vi "compileScript.vi"(8 "error in (no error)":errorcluster, 10 "Path":path, 11 "Compiler in":refnum<class "Compiler.lvclass">) -> (0 "error out":errorcluster, 2 "CompiledList":refnum<class "CompiledList.lvclass">, 3 "Compiler out":refnum<class "Compiler.lvclass">)   [LabVIEW 2011, in "Compiler.lvlib" / "Compiler.lvclass"]
uses:
  Compiler.lvclass
  CompiledList/CompiledList.lvclass
  Compiler.lvclass/Compiler.ctl
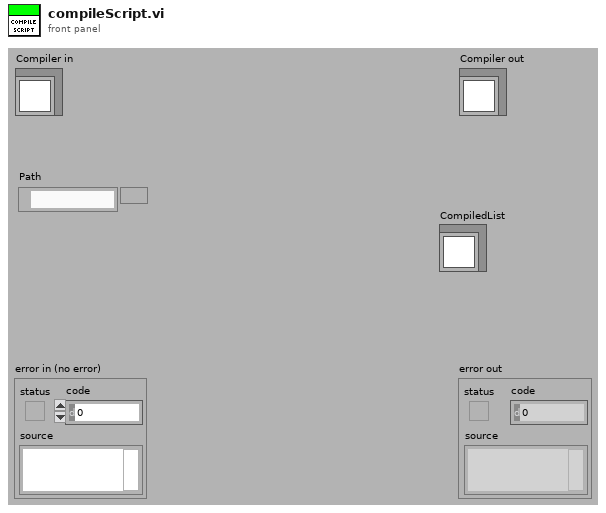
[diagram p1: front panel]
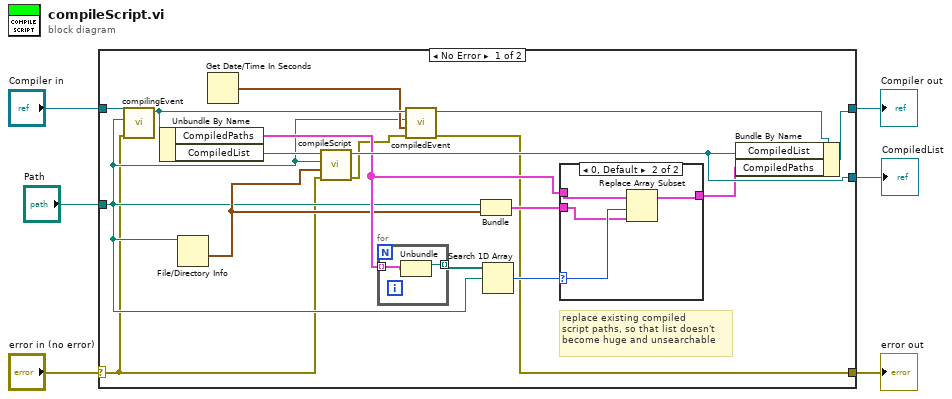
[diagram p0: block diagram]
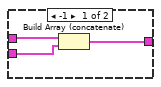
[diagram p2: hidden frame]
diagram:
  n1 = case shown="No Error" "error in (no error)" {
    selector: "error in (no error)" -> [w10 w34]
    tunnel: [w9 w34] -> w5
    tunnel: [w7 w33] -> w3
    tunnel: "Compiler in" -> [w16 w33]
    tunnel: "Path" -> [w11 _]
    tunnel: [w22 _] -> w1
    frame No Error {
      # "replace existing compiled\nscript paths, so that list doesn't\nbecome huge and unsearchable"
      n2 = call "compilingEvent.vi"("error in (no error)"=w10, "Path"=w11, "Compiler in"=w16) -> ("Compiler out"=w15:refnum<class "Compiler.lvclass">)  [unwired: 7 in, 1 out]
      n3 = Unbundle By Name(w15) -> ("CompiledPaths"=w18:cluster{path, "lastCompiled":timestamp}[], "CompiledList"=w23:refnum<class "CompiledList.lvclass">)
      n4 = File/Directory Info(path=w11) -> (last mod=w13:timestamp)  [unwired: 1 in, 6 out]
      n5 = Get Date/Time In Seconds() -> (seconds since 1Jan1904=w12:timestamp)
      n6 = call "compileScript.vi"("error in (no error)"=w10, "current time"=w13, "Path"=w11, "CompiledList in"=w23) -> ("error out"=w14:errorcluster, "CompiledList out"=w22:refnum<class "CompiledList.lvclass">)  [unwired: 6 in]
      n7 = for {
        tunnel: w18 -> [w32] mode=indexing
        tunnel: [w31] -> w21 mode=indexing
        n8 = Unbundle(w32) -> (w31:path)  [unwired: 1 out]
      }
      n9 = call "compiledEvent.vi"("error in (no error)"=w14, "current time"=w12, "Path"=w11, "Compiler in"=w15) -> ("error out"=w9:errorcluster, "Compiler out"=w8:refnum<class "Compiler.lvclass">)  [unwired: 6 in]
      n10 = Bundle("Path"=w11, "last mod"=w13) -> (w20:cluster{"Path":path, "last mod":timestamp})  [unwired: 1 in]
      n11 = Search 1D Array(1D array=w21, element=w11) -> (index of element=w19:i32)  [unwired: 1 in]
      n12 = case shown="0, Default" w19 {
        selector: w19 -> [_ w29]
        tunnel: w20 -> [w25 w28]
        tunnel: w18 -> [w26 w30]
        tunnel: [w24 w27] -> w17
        frame -1 {
          n13 = Build Array (concatenate)(w26, w25) -> (w24:cluster{"Path":path, "last mod":timestamp}[])
        }
        frame 0, Default {
          n14 = Replace Array Subset(array=w30, new element=w28, index=w29) -> (w27:cluster{path, "lastCompiled":timestamp}[])
        }
      }
      n15 = Bundle By Name(cluster=w8, "CompiledList"=w22, "CompiledPaths"=w17) -> (w7:refnum<class "Compiler.lvclass">)
    }
    frame Error {
    }
  }
  "error out" <- w5
  "Compiler out" <- w3
  "CompiledList" <- w1
